vi "Monitor.vi"(8 "error in (no error)":errorcluster, 9 "Channel (0)":u16, 10 "Command (0:On)":u16(ring) items=["On", "Off", "Status", "Read"], 11 "VISA Resource Name":refnum<visa-resource-name>) -> (0 "error out":errorcluster, 1 "Channel?":string, 2 "Channel Output":dbl format="%.2f", 3 "VISA Resource Name Out":refnum<visa-resource-name>, 4 "On/Off?":bool)   [LabVIEW 2012, in "Agilent 34970.lvlib"]
doc: "This VI allows you to use the instrument's monitor mode. You can turn the monitor mode on and monitor a selected channel. You can check the status (on/off) and current channel of the monitor mode. Or, you can turn the monitor mode off."
uses:
  <instrlib>/Agilent 34970/Agilent 34970.lvlib
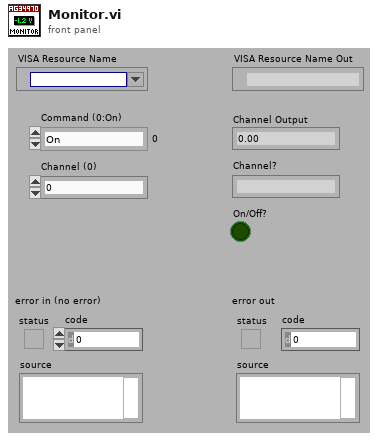
[diagram p1: front panel]
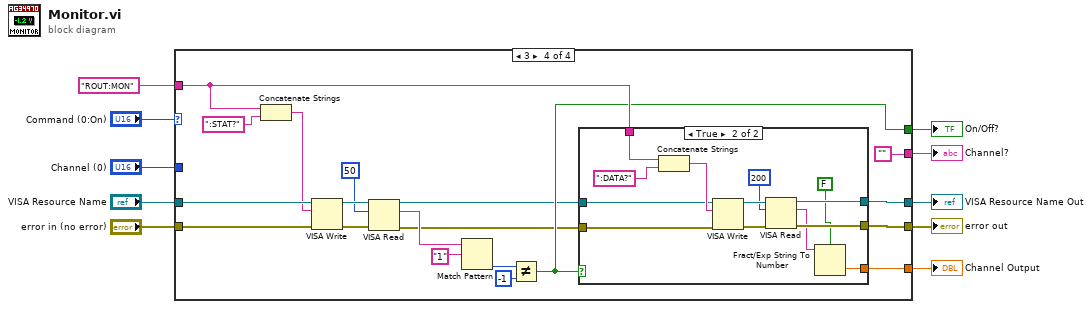
[diagram p0: block diagram]
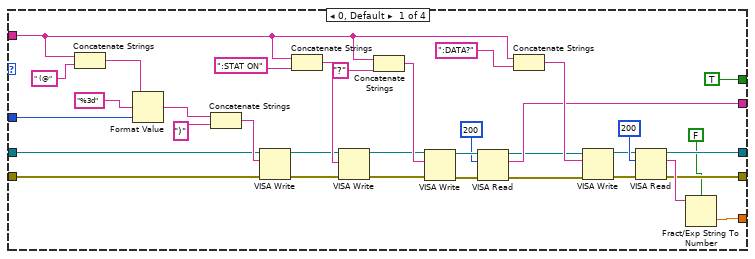
[diagram p2: hidden frame]
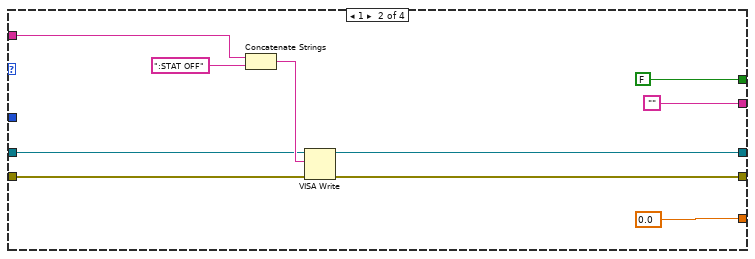
[diagram p3: hidden frame]
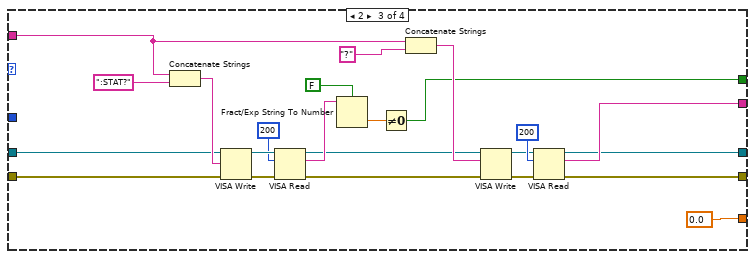
[diagram p4: hidden frame]
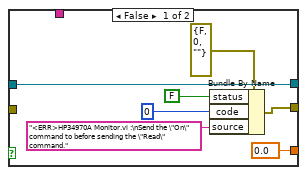
[diagram p5: hidden frame]
diagram:
  n1 = case shown="3" "Command (0:On)" {
    tunnel: "ROUT:MON" ("string (\"\")") -> [w18 w55 w62 w94]
    tunnel: "Channel (0)" -> [w36 _ _ _]
    tunnel: "VISA Resource Name" -> [w35 w52 w76 w92]
    tunnel: "error in (no error)" -> [w34 w51 w75 w91]
    tunnel: [w26 w50 w58 w96] -> w3
    tunnel: [w25 w46 w59 w97] -> w2
    tunnel: [w27 0.0 0.0 w95] -> w7
    tunnel: [TRUE FALSE w61 w82] -> w6
    tunnel: [w15 "" w60 ""] -> w5
    frame 0, Default {
      n2 = Concatenate Strings(w18, " (@") -> (w13:string)
      n3 = Format Value(string ("")=w13, format string="%3d", value (0)=w36) -> (output string=w42:string)
      n4 = Concatenate Strings(w42, ")") -> (w41:string)
      n5 = VISA Write(VISA resource name=w35, write buffer=w41, error in (no error)=w34) -> (VISA resource name out=w38:refnum<visa-resource-name>, error out=w37:errorcluster)  [unwired: 1 out]
      n6 = Concatenate Strings(w18, ":STAT ON") -> (w39:string)
      n7 = VISA Write(VISA resource name=w38, write buffer=w39, error in (no error)=w37) -> (VISA resource name out=w17:refnum<visa-resource-name>, error out=w16:errorcluster)  [unwired: 1 out]
      n8 = Concatenate Strings(w18, "?") -> (w19:string)
      n9 = VISA Write(VISA resource name=w17, write buffer=w19, error in (no error)=w16) -> (VISA resource name out=w22:refnum<visa-resource-name>, error out=w21:errorcluster)  [unwired: 1 out]
      n10 = VISA Read(VISA resource name=w22, byte count=u32 200 ("byte count (0)"), error in (no error)=w21) -> (VISA resource name out=w12:refnum<visa-resource-name>, read buffer=w15:string, error out=w11:errorcluster)  [unwired: 1 out]
      n11 = Concatenate Strings(w18, ":DATA?") -> (w32:string)
      n12 = VISA Write(VISA resource name=w12, write buffer=w32, error in (no error)=w11) -> (VISA resource name out=w29:refnum<visa-resource-name>, error out=w28:errorcluster)  [unwired: 1 out]
      n13 = VISA Read(VISA resource name=w29, byte count=u32 200 ("byte count (0)"), error in (no error)=w28) -> (VISA resource name out=w25:refnum<visa-resource-name>, read buffer=w31:string, error out=w26:errorcluster)  [unwired: 1 out]
      n14 = Fract/Exp String To Number(use system decimal point (T)=FALSE, string=w31) -> (number=w27:dbl)  [unwired: 2 in, 1 out]
    }
    frame 1 {
      n15 = Concatenate Strings(w55, ":STAT OFF") -> (w53:string)
      n16 = VISA Write(VISA resource name=w52, write buffer=w53, error in (no error)=w51) -> (VISA resource name out=w46:refnum<visa-resource-name>, error out=w50:errorcluster)  [unwired: 1 out]
    }
    frame 2 {
      n17 = Concatenate Strings(w62, ":STAT?") -> (w77:string)
      n18 = VISA Write(VISA resource name=w76, write buffer=w77, error in (no error)=w75) -> (VISA resource name out=w74:refnum<visa-resource-name>, error out=w73:errorcluster)  [unwired: 1 out]
      n19 = VISA Read(VISA resource name=w74, byte count=u32 200 ("byte count (0)"), error in (no error)=w73) -> (VISA resource name out=w63:refnum<visa-resource-name>, read buffer=w70:string, error out=w71:errorcluster)  [unwired: 1 out]
      n20 = Fract/Exp String To Number(use system decimal point (T)=FALSE, string=w70) -> (number=w69:dbl)  [unwired: 2 in, 1 out]
      n21 = Not Equal To 0?(x=w69) -> (x != 0?=w61:bool)
      n22 = Concatenate Strings(w62, "?") -> (w68:string)
      n23 = VISA Write(VISA resource name=w63, write buffer=w68, error in (no error)=w71) -> (VISA resource name out=w65:refnum<visa-resource-name>, error out=w66:errorcluster)  [unwired: 1 out]
      n24 = VISA Read(VISA resource name=w65, byte count=u32 200 ("byte count (0)"), error in (no error)=w66) -> (VISA resource name out=w59:refnum<visa-resource-name>, read buffer=w60:string, error out=w58:errorcluster)  [unwired: 1 out]
    }
    frame 3 {
      n25 = Concatenate Strings(w94, ":STAT?" ("write buffer")) -> (w90:string)
      n26 = VISA Write(VISA resource name=w92, write buffer=w90, error in (no error)=w91) -> (VISA resource name out=w89:refnum<visa-resource-name>, error out=w88:errorcluster)  [unwired: 1 out]
      n27 = VISA Read(VISA resource name=w89, byte count=u32 50, error in (no error)=w88) -> (VISA resource name out=w80:refnum<visa-resource-name>, read buffer=w86:string, error out=w79:errorcluster)  [unwired: 1 out]
      n28 = Match Pattern(string=w86, regular expression="1") -> (offset past match=w84:i32)  [unwired: 1 in, 3 out]
      n29 = Not Equal?(x=w84, y=-1) -> (x != y?=w82:bool)
      n30 = case shown="True" w82 {
        tunnel: w94 -> [_ w116]
        tunnel: [w103 w112] -> w97
        tunnel: [w101 w111] -> w96
        tunnel: [0.0 w108] -> w95
        tunnel: w80 -> [w103 w106]
        tunnel: w79 -> [_ w105]
        frame False {
          n31 = Bundle By Name(cluster=errorcluster {"status"=FALSE, "code"=0, "source"=""} ("error out"), "status"=FALSE, "code"=0, "source"="<ERR>HP34970A Monitor.vi :\nSend the \"On\" command to before sending the \"Read\" command.") -> (w101:errorcluster)
        }
        frame True {
          n32 = Concatenate Strings(w116, ":DATA?") -> (w115:string)
          n33 = VISA Write(VISA resource name=w106, write buffer=w115, error in (no error)=w105) -> (VISA resource name out=w114:refnum<visa-resource-name>, error out=w113:errorcluster)  [unwired: 1 out]
          n34 = VISA Read(VISA resource name=w114, byte count=u32 200 ("byte count (0)"), error in (no error)=w113) -> (VISA resource name out=w112:refnum<visa-resource-name>, read buffer=w110:string, error out=w111:errorcluster)  [unwired: 1 out]
          n35 = Fract/Exp String To Number(use system decimal point (T)=FALSE, string=w110) -> (number=w108:dbl)  [unwired: 2 in, 1 out]
        }
      }
    }
  }
  "Channel Output" <- w7
  "On/Off?" <- w6
  "Channel?" <- w5
  "error out" <- w3
  "VISA Resource Name Out" <- w2
